vi "RWA_PC FIle Read String.vi"(8 "Error":errorcluster, 11 "Path":path) -> (0 "Error Out":errorcluster, 1 "Found":bool, 2 "String Out":string, 3 "Duplicate Path Out":path)   [LabVIEW 2020]
uses:
  Error Handling/MGI Suppress Error Code/MGI Suppress Error Code (Scalar).vi
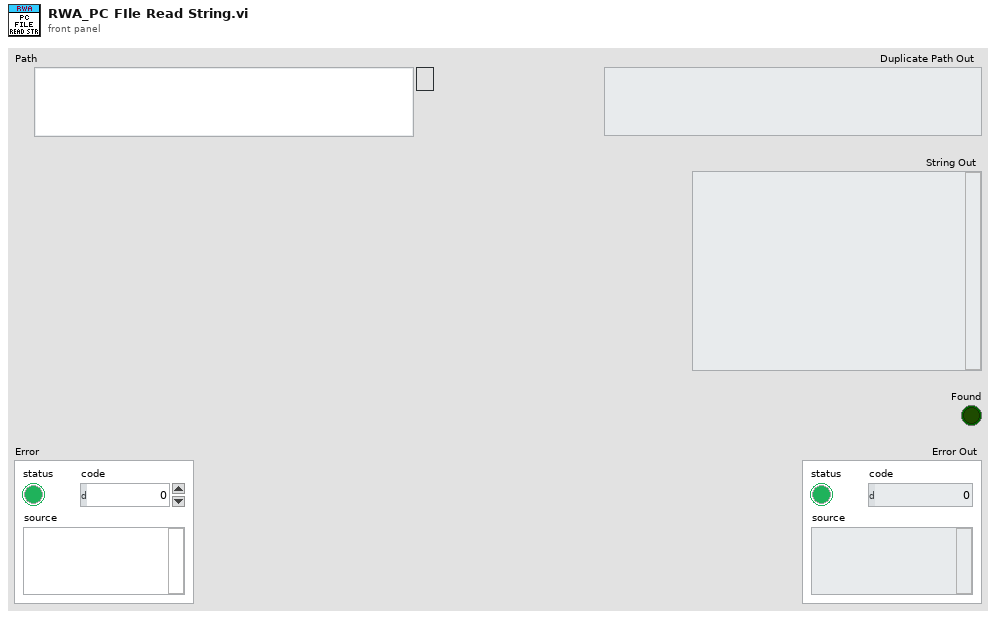
[diagram p1: front panel]
types:
  T1 = enum16{"Auto Detect", "Path Contains a File", "Path Does Not Contain a File"}
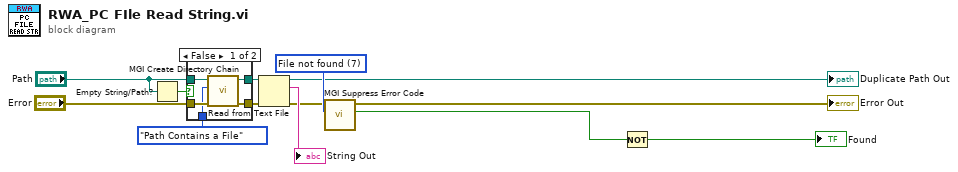
[diagram p0: block diagram]
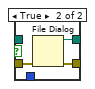
[diagram p2: hidden frame]
diagram:
  w11 = u16 7 items=["No error", "Argument error", "Memory is full", "Out of zone", "End of file", "File already open", "Generic file I/O error", "File not found", "File permission error", "Disk is full", "Duplicate path", "Too many files open", "System feature not enabled", "Resource file not found", "Cannot add resource", "Resource not found", "Image not found", "Image memory error", "Pen does not exist", "Config type invalid", "Config token not found", "Config parse error", "Config memory error", "Bad external code format", "Bad external code offset", "External code not present", "Null window", "Destroy window error", "Null menu", "Print aborted", "Bad print record", "Print driver error", "Windows error during printing", "Memory error during printing", "Print dialog error", "Generic print error", "Invalid device refnum", "Device not found", "Device parameter error", "Device unit error", "Cannot open device", "Device call aborted", "Generic error", "Cancelled by user", "Object ID too low", "Object ID too high", "Object not in heap", "Unknown heap", "Unknown object (invalid DefProc)", "Unknown object (DefProc not in table)", "Message out of range", "Invalid (null) method", "Unknown message", "Manager call not supported", "Bad address", "Network operation in progress", "Network operation timed out", "Connection is busy", "Network attribute not supported", "Network error", "Address in use", "System out of memory", "Connection aborted", "Connection refused", "Not connected", "Already connected", "Connection closed", "Initialization error (interapplication manager)", "Bad occurrence", "Wait on unbound occurrence handler", "Occurrence queue overflow", "Datalog type conflict", "Unused", "Unrecognized type (interapplication manager)", "Memory corrupt", "Failed to make temporary DLL", "Old CIN version", "Drag socket not found", "Failed to load drop-object", "Failed to register OLE object", "Failed to release OLE object", "Format specifier type mismatch", "Unknown format specifier", "Too few format specifiers", "Too many format specifiers", "Scan failed", "Newer CIN version", "OLE Convert", "Runtime menu error", "Password tampered", "Unknown error code"] ("Reserved Error Code (Generic error)")
  n1 = Empty String/Path?(string/path="Path") -> (empty?=w7:bool)
  n2 = case shown="False" w7 {
    tunnel: "Error" -> [w17 w20]
    tunnel: [w16 w19] -> w4
    tunnel: [w15 w18] -> w5
    tunnel: "Path" -> [w14 _]
    tunnel: T1."Path Contains a File" ("File Presence (Auto Detect)") -> [w13 _]
    frame False {
      n3 = call "MGI Create Directory Chain.vi"("Error In"=w17, "File Presence (Auto Detect)"=w13, "Path"=w14) -> ("Error Out"=w16:errorcluster, "Duplicate Path"=w15:path)  [unwired: 7 out]
    }
    frame True {
      n4 = File Dialog(8:w20) -> (0:w19:errorcluster, 3:w18:path)  [unwired: 8 out]
    }
  }
  "Duplicate Path Out" <- w5
  n5 = Read from Text File(file (use dialog)=w5, error in=w4) -> (text=→"String Out":string, error out=w9:errorcluster)  [unwired: 4 out]
  n6 = call-poly "MGI Suppress Error Code.vi"("Error Code"=w11, "Error In"=w9) -> ("Error Supressed?"=w2:bool, "Error Out"=→"Error Out":errorcluster)  [unwired: 4 in]
  n7 = Not(x=w2) -> (.not. x?=→"Found":bool)
